vi "SYST_COMM_GPIB_RDEV_CLOS.vi"(0 "VISA IN":refnum<visa-resource-name>, 5 "error in":errorcluster, 7 "ID":i32) -> (14 "VISA Out":refnum<visa-resource-name>, 19 "error out":errorcluster)   [LabVIEW 2018, in "PNA-X.lvlib"]
doc: "SYSTem:COMMunicate:GPIB:RDEVice:CLOSe <ID> \n1869\n\n(Write only) Closes the remote GPIB session. This command should be sent when ending every \nsuccessful OPEN session. \nParameters \n<ID> Session identification number that was returned with the OPEN? command. \nExamples See an example program \nQuery Syntax Not Applicable \nDefault Not Applicable"
uses:
  PNA-X.lvlib
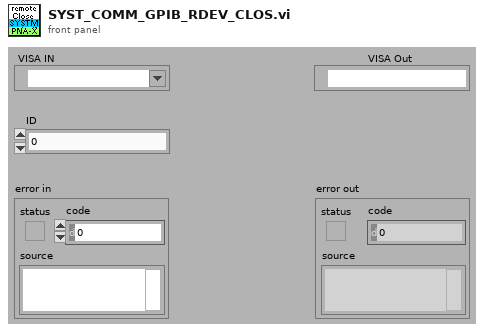
[diagram p1: front panel]
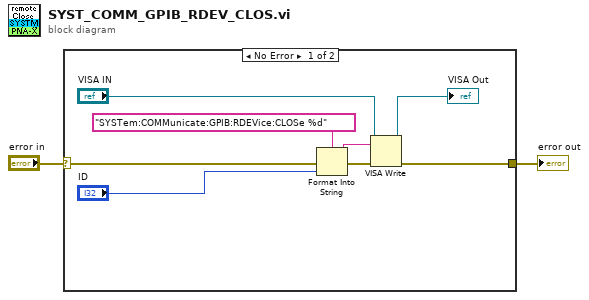
[diagram p0: block diagram]
diagram:
  n1 = case shown="No Error" "error in" {
    selector: "error in" -> [w10 w11]
    tunnel: [w5 w11] -> w1
    frame No Error {
      n2 = Format Into String(format string="SYSTem:COMMunicate:GPIB:RDEVice:CLOSe %d" ("Cmdline"), error in=w10, "ID") -> (resulting string=w8:string, error out=w9:errorcluster)  [unwired: 1 in]
      n3 = VISA Write(VISA resource name="VISA IN", write buffer=w8, error in (no error)=w9) -> (VISA resource name out=→"VISA Out":refnum<visa-resource-name>, error out=w5:errorcluster)  [unwired: 1 out]
    }
    frame Error {
    }
  }
  "error out" <- w1
